vi "tkrsa6100 Error Info Parser.vi"(11 "Input String":string) -> (1 "Error Status":bool, 2 "Error #":i32, 3 "Response String":string)   [LabVIEW 2020, in "Library Instrument & Equipement.lvlib" / "Library Spectrum Analyser.lvlib"]
doc: "This VI parses the remaining instrument response after the error information string is removed into the actual instrument response and updates the error out cluster's error code and error # information.\n\nThe format of the input string is:\n\n<,0;9+E0000000000.1> which is the reversed version of <1.00000000000E+9;0,>\n\nThe first semicolon in the reversed string (which separates the instrument query response and the error information) is detected with a Match Pattern function.\n\nThe after substring output passes the instrument response to string indicator Response String after the string is again reversed to get it into its correct order.\n\nThe before substring output passes the error # to another Match Pattern function which detects the leading comma. The after substring output passes the error number without the comma to another reverse string function which gets it back into its correct order.\n\nThe error number string is converted to a numeric which updates indicator Error #. If Error # is 0, indicator Error Status is set to False. Otherwise it is set to True."
uses:
  Library Spectrum Analyser.lvlib
panel:
  # "Error String Parser"
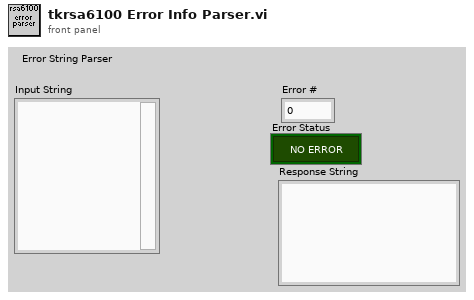
[diagram p1: front panel]
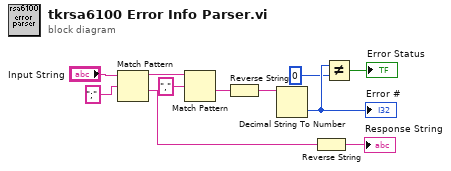
[diagram p0: block diagram]
diagram:
  n1 = Match Pattern(string="Input String", regular expression=";") -> (before substring=w3:string, after substring=w1:string)  [unwired: 3 out]
  n2 = Match Pattern(string=w3, regular expression=",") -> (after substring=w4:string)  [unwired: 4 out]
  n3 = Reverse String(1:w4) -> (0:w5:string)
  n4 = Decimal String To Number(string=w5) -> (number=w10:i32)  [unwired: 3 out]
  "Error #" <- w10
  n5 = Reverse String(1:w1) -> (0:→"Response String":string)
  n6 = Not Equal?(x=w10, y=0) -> (x != y?=→"Error Status":bool)
